vi "Handle Enable Disable Key Down Events.vi"(6 "UI Event Regs in":T1, 7 "Owning VI":refnum<vi>, 8 "error in (no error)":errorcluster, 11 "Enable/Disable":bool) -> (0 "error out":errorcluster, 4 "UI Event Regs out":T1)   [LabVIEW 2020, in "AR Example.lvlib" / "UI.lvclass"]
uses:
  UI.lvclass
  UI.lvclass/UI.ctl
  Stop Event.ctl
  g_ar_toolkit.image/Image Draw Offset.ctl
  g_ar_toolkit.image/g_ar_toolkit.image.lvlib
  Update Preview Event.ctl
  Events.ctl
  UI Event Registrations.ctl
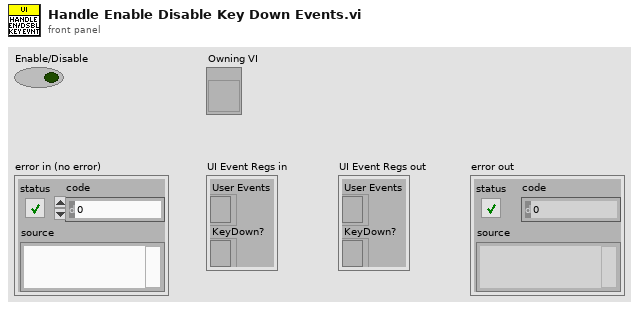
[diagram p1: front panel]
types:
  T1 = typedef "AR Example.lvlib/UI.lvclass/UI Event Registrations.ctl" = cluster{"User Events":refnum<event-registration>, "KeyDown?":refnum<event-registration>}
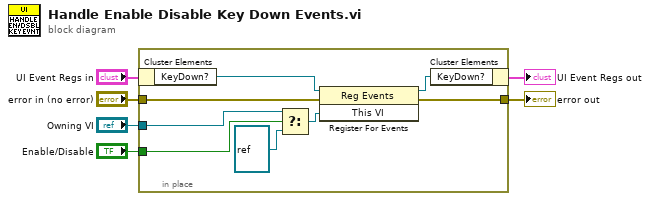
[diagram p0: block diagram]
diagram:
  n1 = in-place {
    in-place-border: "Enable/Disable" -> [w12]
    in-place-border: "Owning VI" -> [w10]
    in-place-border: "error in (no error)" -> [w9]
    in-place-border: [w8] -> w1
    n2 = in-place-cluster #1("UI Event Regs in") -> ("KeyDown?"=w14:refnum<event-registration>)
    n3 = Select(t=w10, s=w12, f=refnum<vi> refnum) -> (s? t:f=w11:refnum<vi>)
    n4 = register-events(reference=w14, error in=w9, w11) -> (reference out=w13:refnum<event-registration>, error out=w8:errorcluster)
    n5 = in-place-cluster #1("KeyDown?"=w13) -> (→"UI Event Regs out":T1)
  }
  "error out" <- w1
